vi "Mercury_GoToField_SubVI.vi"(8 "error in (no error)":errorcluster, 11 "Targets":T1) -> (0 "error out":errorcluster)   [LabVIEW 2016, in "Instrument.OxfordVRM.lvclass"]
doc: "USE AT YOUR OWN RISK!\nThis subVI is meant to be called as a subVI of \"Mercury_GoToField.vi\", which will take care of the persistent switch for you"
uses:
  Instrument.OxfordVRM.lvclass
  Typedefs/VRM Targets--Cluster.ctl
  <userlib>/LevyLab/Levylab Instruments/Instrument Types/Cryostat/Typedefs/VRM Magnet Axis--Enum.ctl
panel:
  # "USE AT YOUR OWN RISK!\nThis subVI is meant to be called as a subVI of \"Mercury_GoToField.vi\", which will take care of the persistent switch for you"
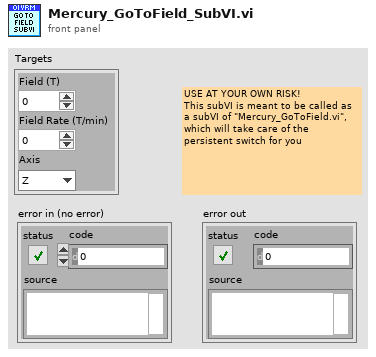
[diagram p1: front panel]
types:
  T1 = typedef "Instrument.OxfordVRM.lvclass/VRM Targets--Cluster.ctl" = cluster{"Field (T)":dbl, "Field Rate (T/min)":dbl, "Axis":T2}
  T2 = typedef "Instrument.OxfordVRM.lvclass/VRM Magnet Axis--Enum.ctl" = enum16{"Z", "X", "Y", "ALL"}
  T3 = typedef "Instrument.OxfordVRM.lvclass/Actions.ctl" = cluster{"Hold":bool, "Clamp":bool, "To Set":bool, "To Zero":bool, "Send to IPS":bool, "PS Heat":bool, "Lambda":bool}
  T4 = typedef "Instrument.OxfordVRM.lvclass/Status.ctl" = cluster{"Magnet Field":dbl, "PS Field":dbl, "Target Field":dbl, "Target Field Rate":dbl, "Voltage":dbl, "Current":dbl, "Switch":bool, "Mercury State":string}
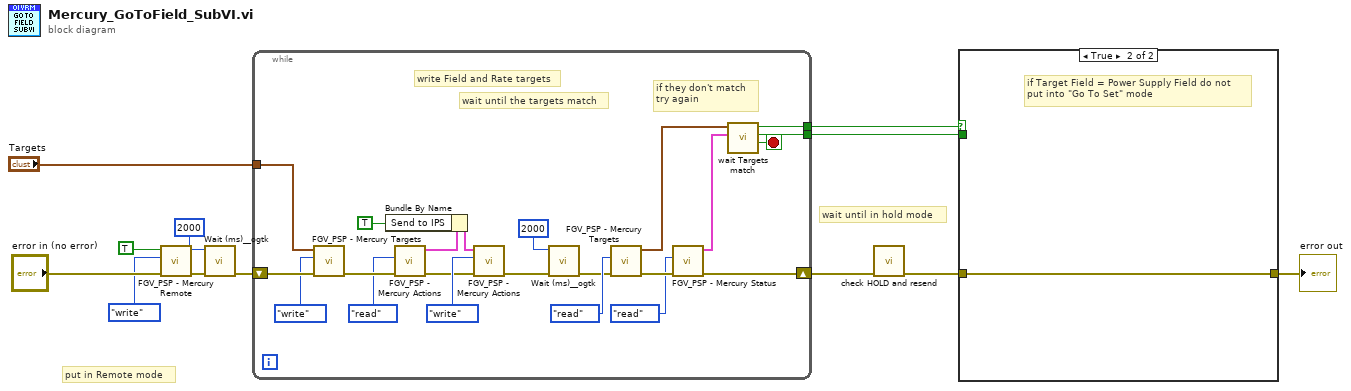
[diagram p0: block diagram]
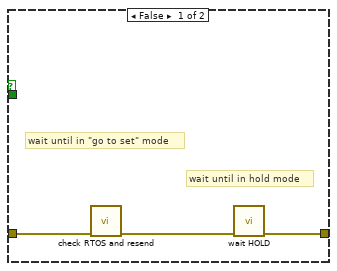
[diagram p2: hidden frame]
diagram:
  # "put in Remote mode"
  # "wait until in hold mode"
  n1 = call "FGV_PSP - Mercury Remote.vi"("error in"="error in (no error)", "Function"=enum16{"write", "read"}."write", "Remote"=TRUE ("Mercury Remote")) -> ("error out"=w5:errorcluster)  [unwired: 3 in, 1 out]
  n2 = call <userlib>:"Wait (ms)__ogtk.vi"("error in (no error)"=w5, "milliseconds to wait"=u32 2000) -> ("error out"=w7:errorcluster)  [unwired: 8 in, 1 out]
  n3 = while {
    tunnel: [w30] -> w11
    tunnel: [w33] -> w10
    shift-right: [w19] -> w9
    shift-left: w7 -> [w29]
    tunnel: "Targets" -> [w26]
    stop <- w32 stop-if-true
    # "if they don't match\ntry again"
    # "wait until the targets match"
    # "write Field and Rate targets"
    n4 = call "FGV_PSP - Mercury Targets.vi"("error in"=w29, "Function"=enum16{"write", "read"}."write", "Targets"=w26) -> ("error out"=w28:errorcluster)  [unwired: 3 in, 1 out]
    n5 = call "FGV_PSP - Mercury Actions.vi"("error in"=w28, "Function"=enum16{"write", "read"}."read") -> ("error out"=w23:errorcluster, "Actions"=w24:T3)  [unwired: 4 in]
    n6 = Bundle By Name(cluster=w24, "Send to IPS"=TRUE) -> (w22:T3)
    n7 = call "FGV_PSP - Mercury Actions.vi"("error in"=w23, "Function"=enum16{"write", "read"}."write", "Actions"=w22) -> ("error out"=w14:errorcluster)  [unwired: 3 in, 1 out]
    n8 = call <userlib>:"Wait (ms)__ogtk.vi"("error in (no error)"=w14, "milliseconds to wait"=u32 2000) -> ("error out"=w13:errorcluster)  [unwired: 8 in, 1 out]
    n9 = call "FGV_PSP - Mercury Targets.vi"("error in"=w13, "Function"=enum16{"write", "read"}."read") -> ("error out"=w20:errorcluster, "Targets"=w21:T1)  [unwired: 4 in]
    n10 = call "FGV_PSP - Mercury Status.vi"("error in"=w20, "Function"=enum16{"write", "read"}."read") -> ("error out"=w19:errorcluster, "Status"=w18:T4)  [unwired: 4 in]
    n11 = call "wait Targets match.vi"("status"=w18, "Mercury Targets"=w21) -> ("Target AND Rate Match"=w32:bool, "Target ~ Magnet"=w33:bool, "Target ~ PS"=w30:bool)  [unwired: 7 in]
  }
  n12 = call "check HOLD and resend.vi"("error in"=w9) -> ("error out"=w1:errorcluster)  [unwired: 10 in]
  n13 = case shown="True" w11 {
    tunnel: [w37 w38] -> w12
    tunnel: w1 -> [w35 w38]
    tunnel: w10 -> [_ _]
    frame False {
      # "wait until in hold mode"
      # "wait until in \"go to set\" mode"
      n14 = call "check RTOS and resend.vi"("error in"=w35) -> ("error out"=w36:errorcluster)  [unwired: 10 in]
      n15 = call "wait HOLD.vi"("error in (no error)"=w36) -> ("error out"=w37:errorcluster)  [unwired: 10 in]
    }
    frame True {
      # "if Target Field = Power Supply Field do not\nput into \"Go To Set\" mode"
    }
  }
  "error out" <- w12
